vi "Destroy Reader Endpoint.vi"(8 "error in (no error)":errorcluster, 11 "Stream in":refnum<class "Stream.lvclass">) -> (0 "error out":errorcluster, 3 "Stream out":refnum<class "Stream.lvclass">)   [LabVIEW 2018, in "Stream.lvclass"]
uses:
  Stream.lvclass
  Stream.lvclass/Stream.ctl
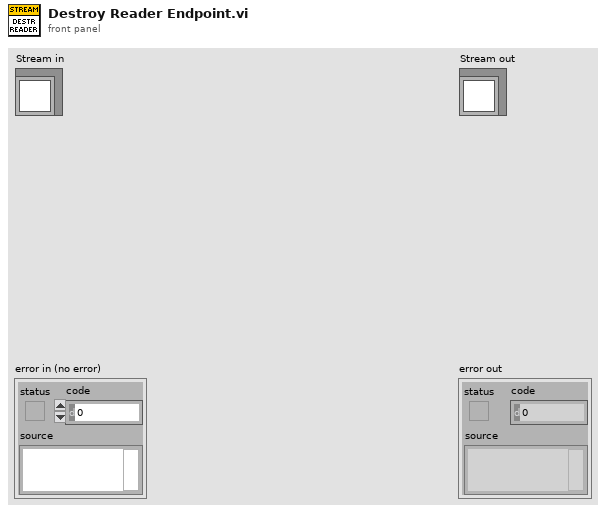
[diagram p1: front panel]
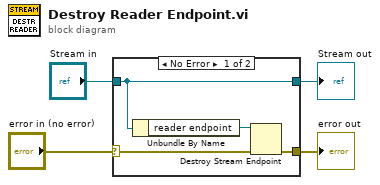
[diagram p0: block diagram]
diagram:
  n1 = case shown="No Error" "error in (no error)" {
    selector: "error in (no error)" -> [w6 w10]
    tunnel: [w7 w10] -> w3
    tunnel: [w8 w9] -> w1
    tunnel: "Stream in" -> [w8 w9]
    frame No Error {
      n2 = Unbundle By Name(w8) -> ("reader endpoint"=w5:refnum<k21>)
      n3 = Destroy Stream Endpoint(8:w6, 11:w5) -> (0:w7:errorcluster)
    }
    frame Error {
    }
  }
  "error out" <- w3
  "Stream out" <- w1
